vi "Solve Polynomial.vi"(8 "error in":errorcluster, 9 "Independants":dbl[](array[numeric]), 10 "Coefficients":dbl[](array[numeric])) -> (0 "error out":errorcluster, 2 "Dependants":dbl[](array[numeric]))   [LabVIEW 2019]
doc: "This VI is designed to calculate a set of independant values given the the coefficients of a polynomial equation. For each dependant value \"x\", the independant \"f(x)\" is determined.\n\nf(x) = a0 + a1*x + a2*x^2 + a3*x^3 ...\n\nAfter using the \"Curve Fit\" Express VI to determine polynomial coefficients, this one can be used to find points along the curve."
panel:
  # "Inputs"
  # "Outputs"
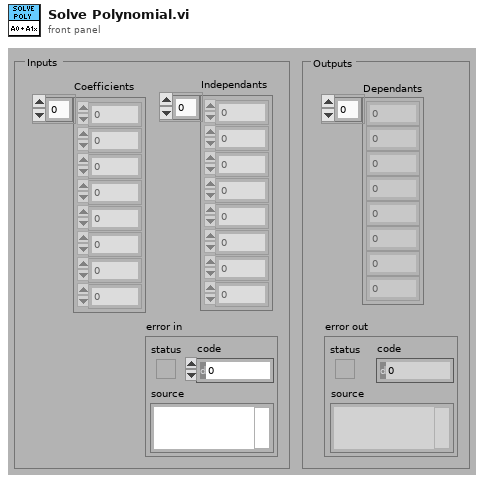
[diagram p1: front panel]
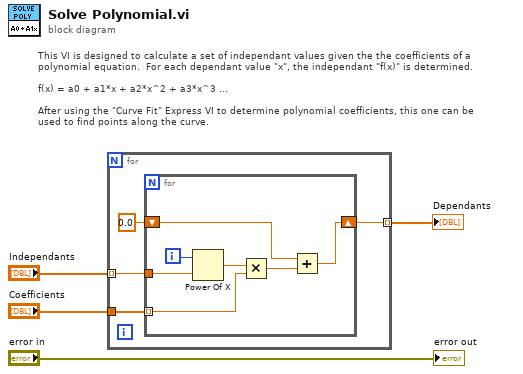
[diagram p0: block diagram]
diagram:
  # "This VI is designed to calculate a set of independant values given the the coefficients of a\npolynomial equation.  For each dependant value \"x\", the independant \"f(x)\" is determined.\n\nf(x) = a0 + a1*x + a2*x^2 + a3*x^3 ...\n\nAfter using the \"Curve Fit\" Express VI to determine polynomial coefficients, this one can be\nused to find points along the curve."
  n1 = for {
    tunnel: "Coefficients" -> [w8]
    tunnel: "Independants" -> [w7] mode=indexing
    tunnel: [w5] -> w2 mode=indexing
    n2 = for {
      tunnel: w8 -> [w12] mode=indexing
      tunnel: w7 -> [w14]
      shift-right: [w9] -> w5
      shift-left: 0.0 -> [w10]
      i -> [w15]
      n3 = Power Of X(1:w14, 2:w15) -> (0:w13:dbl)
      n4 = Multiply(x=w13, y=w12) -> (x*y=w11:dbl)
      n5 = Add(x=w10, y=w11) -> (x+y=w9:dbl)
    }
  }
  "Dependants" <- w2
  "error out" <- "error in"
